vi "Execute New VI From Template.vi"(6 "Mouse Position":T2, 8 "User VI Ref":refnum<vi>, 9 "Menu Item Tag Suffix":string, 10 "Remaining Items":refnum<vi>[](array[refnum]), 11 "Affected Items":cluster{"Any Refnums":refnum<vi>[]}) -> (0 "Fail transaction?":bool)   [LabVIEW 2021]
doc: "This is the main VI of the \"New VI From Template\" shortcut menu plugin.\n\nNotes from shortcut menu template VI:\n1. This VI has no need for a Close Reference call because GObject refnums do not hold the VI in memory. The User VI Ref will be closed by the caller.\n2. You may enable debugging on this VI to help develop your code. Debugging only has to be disabled on the builder VI, not the execute VI.\n\nPetru Tarabuta, Robusto Systems, September 2022"
uses:
  <vilib>/Utility/miscctls.llb/LVPositionTypeDef.ctl
  Owner Status (enum).ctl
  GUI Objects (cluster).ctl
  Testing Flag (enum).ctl
  Testing Flag (library variable).vi
panel:
  in  "SCL":i32(listbox) caption="Templates"
  in  "Apply Owner Icon Template?":bool
  out "Error Out":errorcluster
  out "Owner Filename (including extension)":string
  out "User VI Owner Status":T1
  out "Owner Path":path
  out "Iteration":i32
  out "Tab":enum32{"SomeTemplatesFound", "NoTemplatesFound"}(tab)
  in  "Create":bool
  in  "Destination Location":path
  in  "Add To Owner?":bool caption="Add to Library 1.lvlib?"
  in  "Add To Project?":bool caption="Add to Project?"
  in  "Open Front Panel?":bool caption="Open Front Panel When Created?"
  in  "Project ComboBox":string(combo) caption="Project"
  out "NoTemplatesFound Message":string
  in  "Front Panel Sizing Tool":bool
  # "Execute VI"
  # "The section below is not user-facing. For developer use only."
  # "All controls on this panel except \"Affected Items\" have been locked to prevent accidental edits. Changing the control names or types, other than the elements of the \"Affected Items\" cluster will make the VI unusable as a menu plugin.\n\nSee Context Help for each control for details about its use."
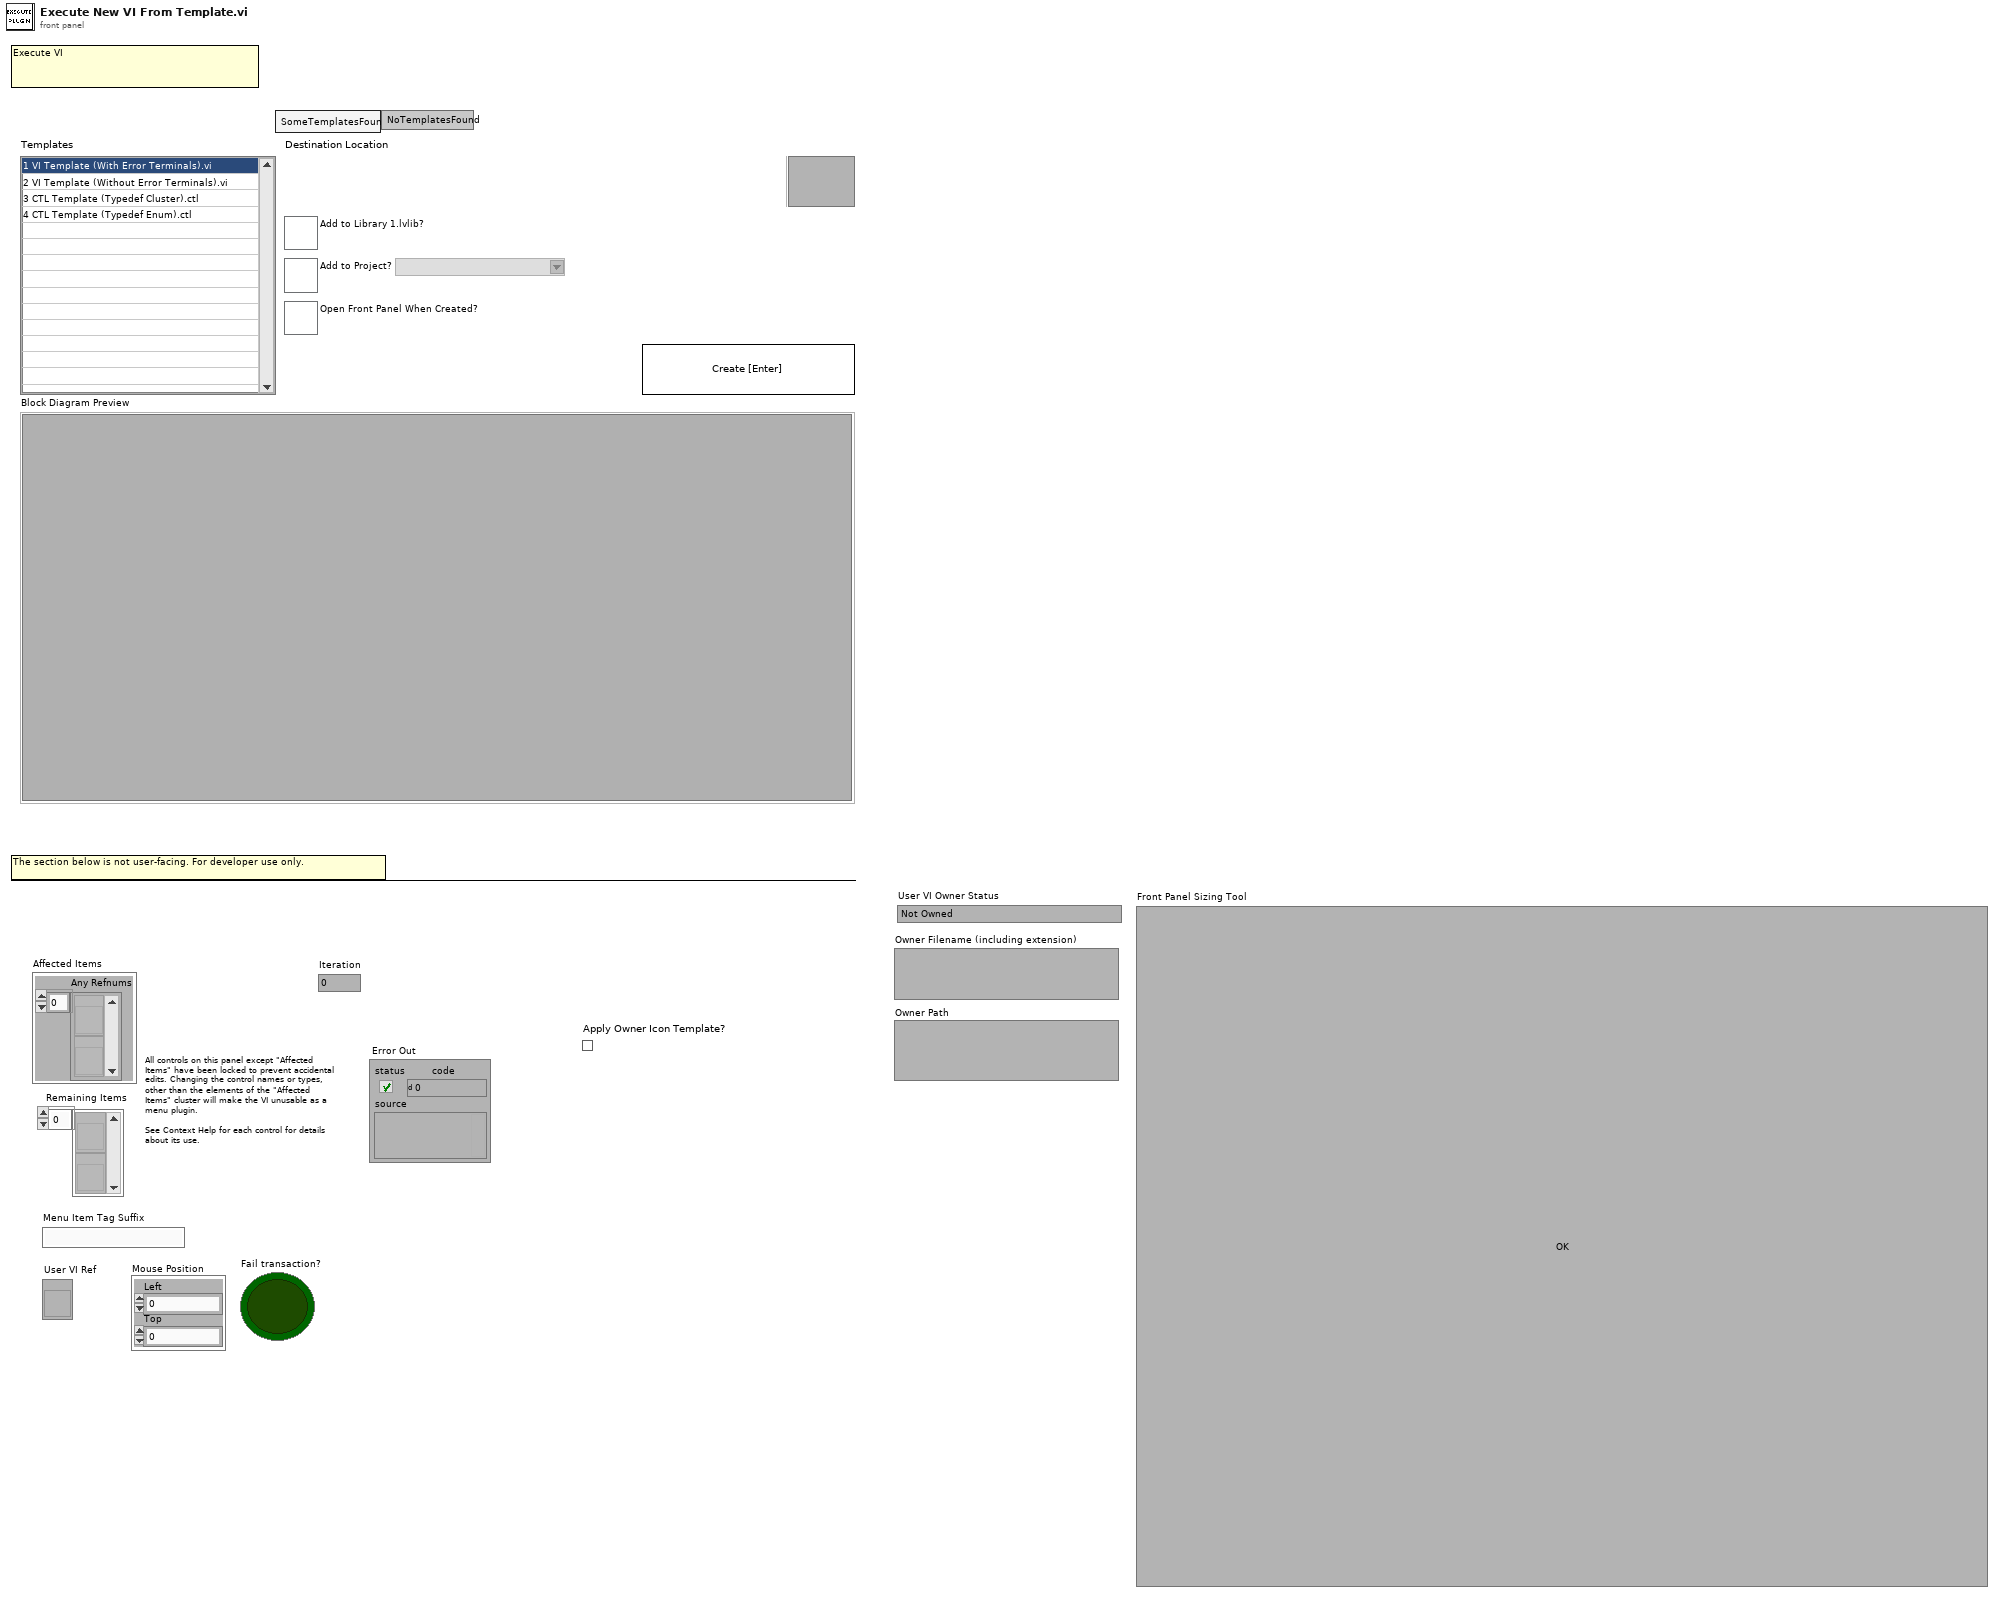
[diagram p1: front panel]
types:
  T1 = typedef "Owner Status (enum).ctl" = enum16{"Not Owned", "Owned by Library (lvlib)", "Owned by Class (lvclass)"}
  T2 = typedef "LVPositionTypeDef.ctl" = cluster{"Left":i32, "Top":i32}
  T3 = typedef "GUI Objects (cluster).ctl" = cluster{"SCL":refnum<vi>, "Add To Owner?":refnum<vi>, "Add To Project?":refnum<vi>, "Open Front Panel?":refnum<vi>, "Destination Folder":refnum<vi>, "Create":refnum<vi>, "Project ComboBox":refnum<vi>, "NoTemplatesFound Message":refnum<vi>, "Diagram Preview Subpanel":refnum<vi>}
  T4 = typedef "Testing Flag (enum).ctl" = enum16{"Production", "Testing"}
  T5 = enum32{"Invalid", "Standard", "Closed", "Hidden", "Minimized", "Maximized"}
  T6 = enum8{"Enabled", "Disabled", "Disabled and Grayed Out"}
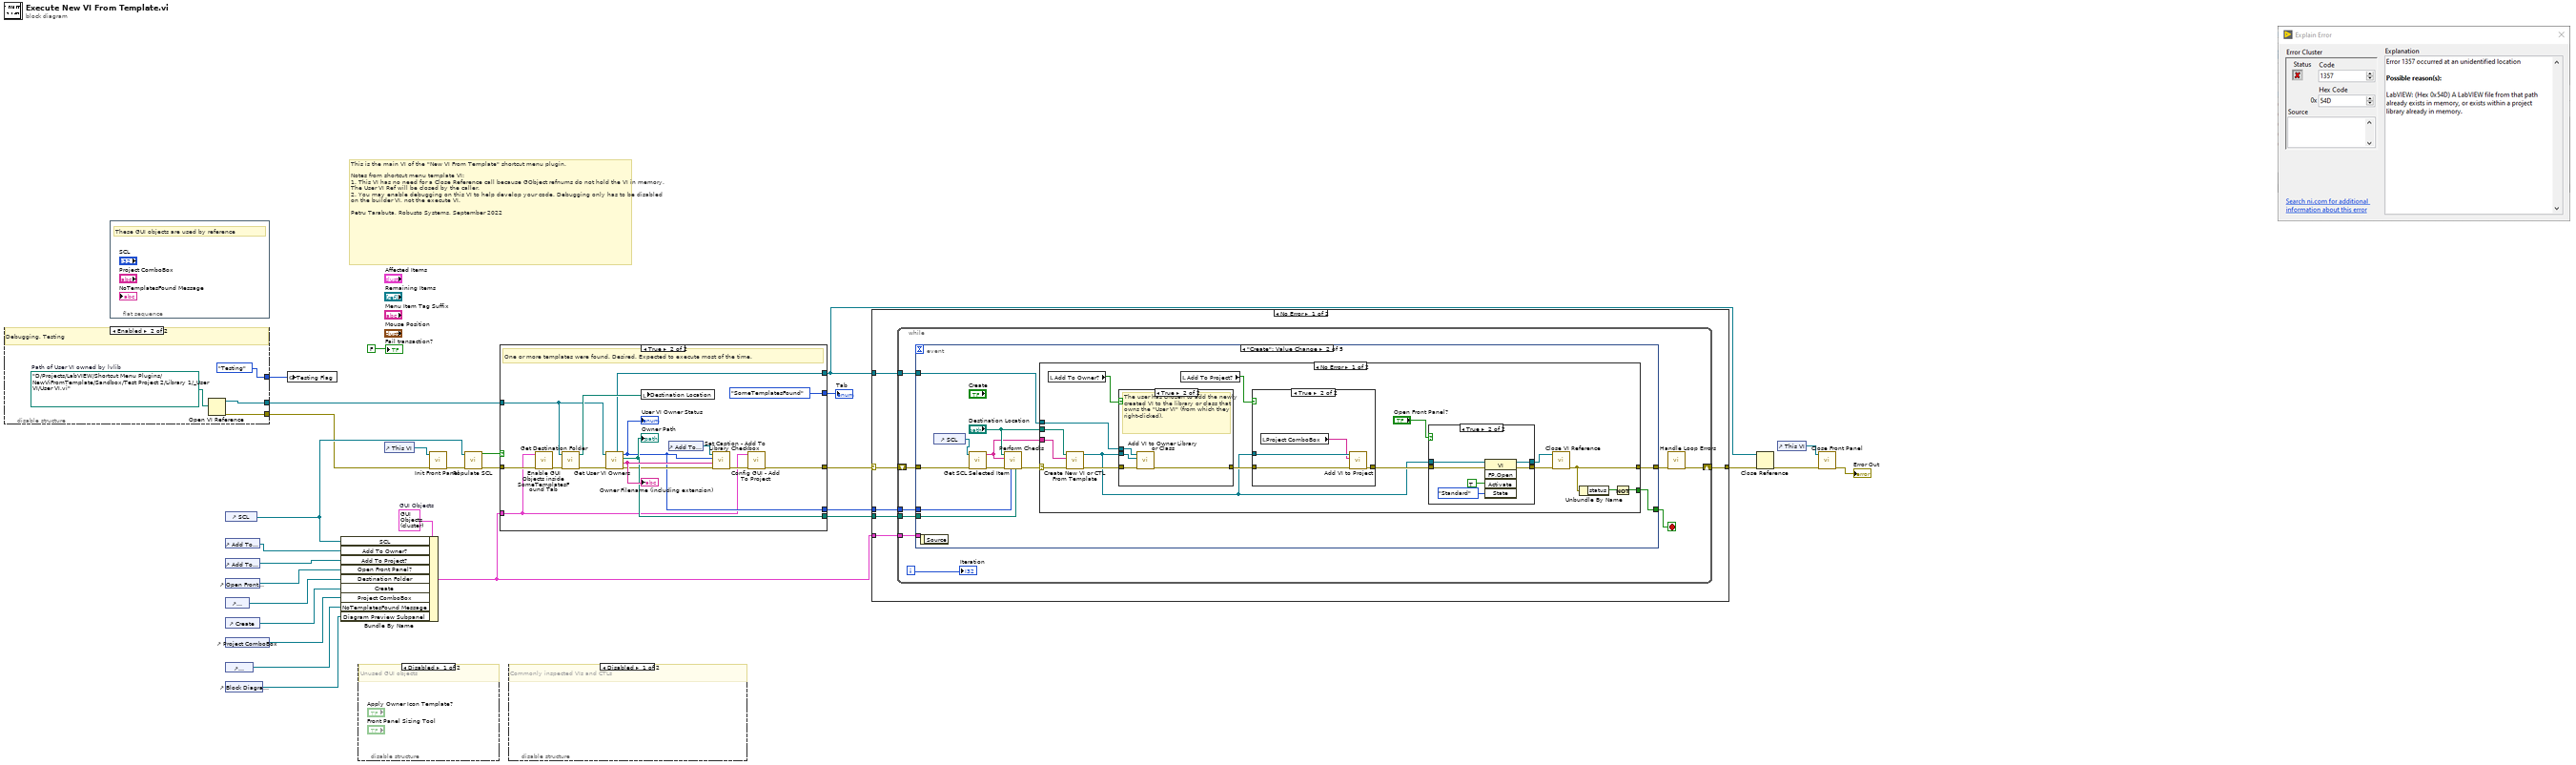
[diagram p0: block diagram]
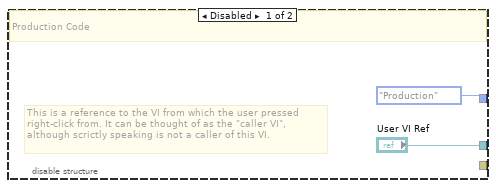
[diagram p3: hidden frame]
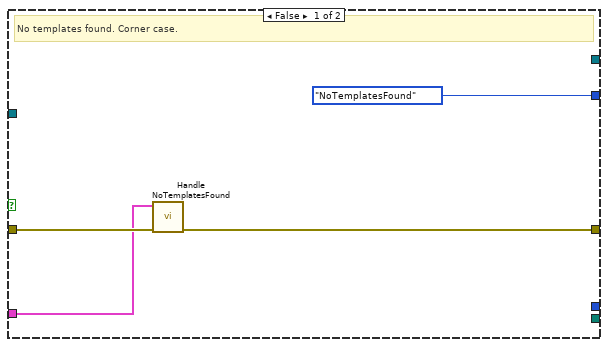
[diagram p4: hidden frame]
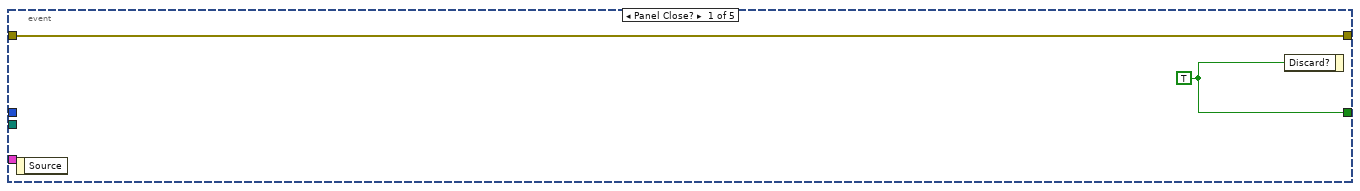
[diagram p6: hidden frame]
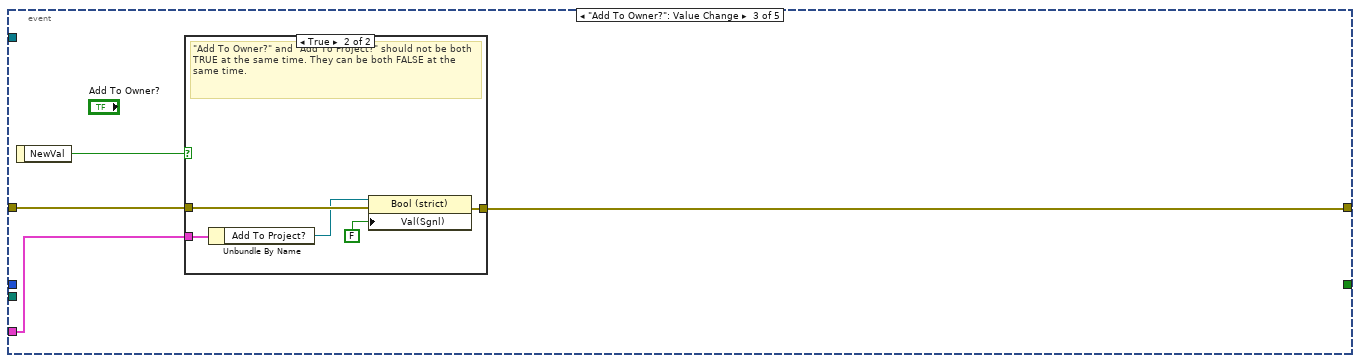
[diagram p11: hidden frame]
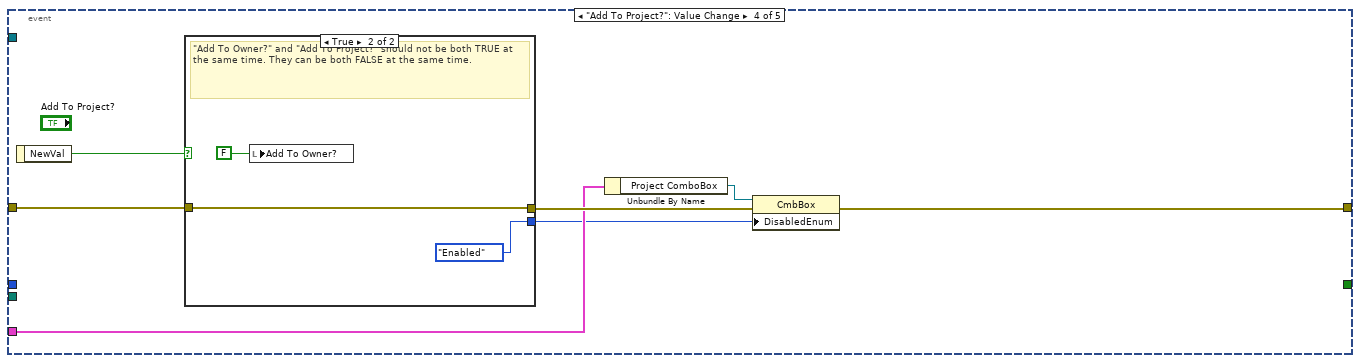
[diagram p13: hidden frame]
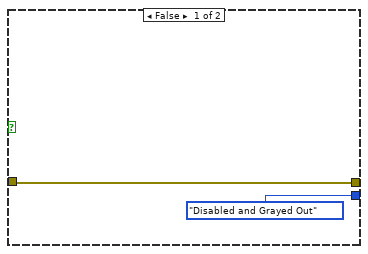
[diagram p14: hidden frame]
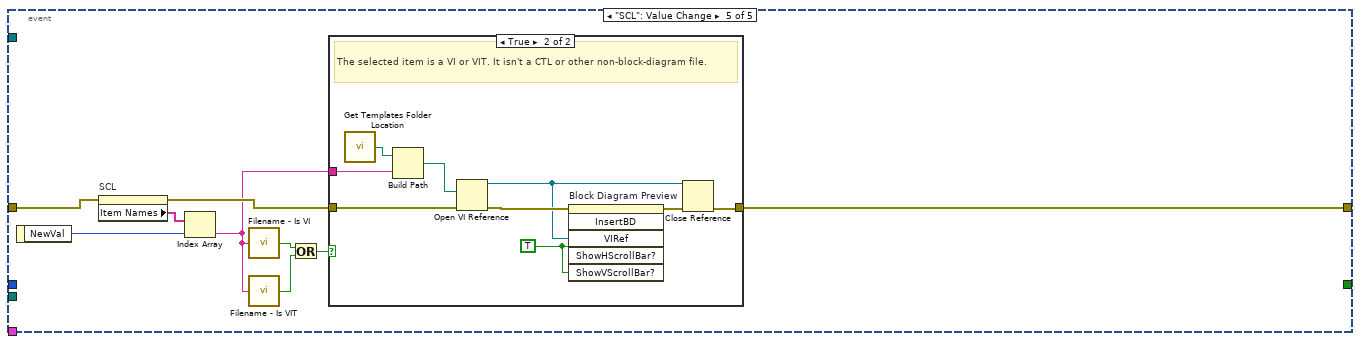
[diagram p15: hidden frame]
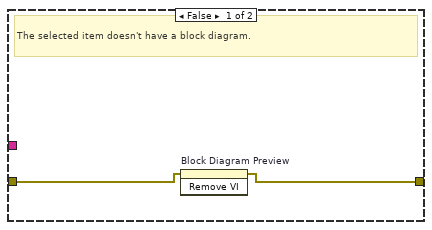
[diagram p16: hidden frame]
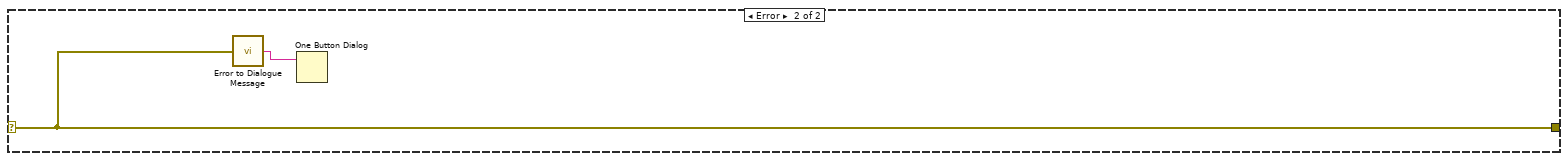
[diagram p17: hidden frame]
diagram:
  w21 = T3 {"SCL"=refnum, "Add To Owner?"=refnum, "Add To Project?"=refnum, "Open Front Panel?"=refnum, "Destination Folder"=refnum, "Create"=refnum, "Project ComboBox"=refnum, "NoTemplatesFound Message"=refnum, "Diagram Preview Subpanel"=refnum}  # GUI Objects
  # "This is the main VI of the \"New VI From Template\" shortcut menu plugin.\n\nNotes from shortcut menu template VI:\n1. This VI has no need for a Close Reference call because GObject refnums do not hold the VI in memory. The User VI Ref will be closed by the caller.\n2. You may enable debugging on this VI to help develop your code. Debugging only has to be disabled on the builder VI, not the execute VI.\n\nPetru Tarabuta, Robusto Systems, September 2022"
  n1 = disable-structure shown="Enabled" {
    disable-tunnel: ["User VI Ref" w32] -> w2
    disable-tunnel: [Testing_Flag_(enum)."Production" ("Testing Flag") Testing_Flag_(enum)."Testing" ("Testing Flag")] -> w12
    disable-tunnel: [_ w31] -> w9
    frame Disabled {
      # "This is a reference to the VI from which the user pressed right-click from. It can be thought of as the \"caller VI\", although scrictly speaking is not a caller of this VI."
      # "Production Code"
    }
    frame Enabled {
      w33 = path "D:/Projects/LabVIEW/Shortcut Menu Plugins/NewViFromTemplate/Sandbox/Test Project 2/Library 1/_User VI/User VI.vi"  # Path of User VI owned by lvlib
      # "Debugging, Testing"
      n2 = Open VI Reference(vi path=w33) -> (vi reference=w32:refnum<vi>, error out=w31:errorcluster)  [unwired: 5 in]
    }
  }
  n3 = flat-sequence {
    frame #0 {
      # "These GUI objects are used by reference"
    }
  }
  n4 = control-ref of="SCL"() -> (w20:refnum<vi>)
  n5 = control-ref of="Add To Owner?"() -> (w19:refnum<vi>)
  n6 = control-ref of="Add To Project?"() -> (w16:refnum<vi>)
  n7 = control-ref of="Open Front Panel?"() -> (w15:refnum<vi>)
  n8 = control-ref of="Destination Location"() -> (w18:refnum<vi>)
  n9 = control-ref of="Create"() -> (w17:refnum<vi>)
  n10 = control-ref of="Project ComboBox"() -> (w8:refnum<vi>)
  n11 = control-ref of="NoTemplatesFound Message"() -> (w3:refnum<vi>)
  n12 = control-ref of="Block Diagram Preview"() -> (w1:refnum<vi>)
  n13 = global write "Testing Flag (library variable).vi" "Testing Flag"(w12) -> ()
  n14 = Bundle By Name(cluster=w21, "SCL"=w20, "Add To Owner?"=w19, "Add To Project?"=w16, "Open Front Panel?"=w15, "Destination Folder"=w18, "Create"=w17, "Project ComboBox"=w8, "NoTemplatesFound Message"=w3, "Diagram Preview Subpanel"=w1) -> (w6:T3)
  n15 = disable-structure shown="Disabled" {
    frame Disabled {
      # "Unused GUI objects"
    }
    frame Enabled {
    }
  }
  n16 = control-ref of="This VI"() -> (w27:refnum<vi>)
  n17 = call "Init Front Panel.vi"("error in"=w9, "VI Reference"=w27) -> ("error out"=w26:errorcluster)  [unwired: 9 in]
  n18 = call "Populate SCL.vi"("error in"=w26, "SCL"=w20) -> ("error out"=w14:errorcluster, "At least one template file found?"=w5:bool)  [unwired: 8 in]
  n19 = case shown="True" w5 {
    tunnel: [_ w48] -> w22
    tunnel: w2 -> [_ w47]
    tunnel: w14 -> [w38 w45]
    tunnel: [_ w44] -> w13
    tunnel: [_ w43] -> w10
    tunnel: [w36 w42] -> w7
    tunnel: w6 -> [w35 w39]
    tunnel: [enum32{"SomeTemplatesFound", "NoTemplatesFound"}."NoTemplatesFound" ("Tab") enum32{"SomeTemplatesFound", "NoTemplatesFound"}."SomeTemplatesFound" ("Tab")] -> w4
    frame False {
      # "No templates found. Corner case."
      n20 = call "Handle NoTemplatesFound.vi"("error in"=w38, "GUI Objects"=w35) -> ("error out"=w36:errorcluster)  [unwired: 9 in]
    }
    frame True {
      # "One or more templates were found. Desired. Expected to execute most of the time."
      n21 = call "Enable GUI Objects inside SomeTemplatesFound Tab.vi"("error in"=w45, "GUI Objects"=w39) -> ("error out"=w40:errorcluster)  [unwired: 9 in]
      n22 = call "Get Destination Folder.vi"("error in"=w40, "User VI Ref"=w47) -> ("error out"=w53:errorcluster, "Destination Folder"=w49:path)  [unwired: 8 in]
      n23 = call "Get User VI Owners.vi"("error in"=w53, "User VI Ref"=w47) -> ("error out"=w46:errorcluster, "Owner Filename (inc file extension)"=w50:string, "Owner Path"=w48:path, "User VI Owner Status"=w44:T1, "Owner Reference"=w43:refnum<vi>)  [unwired: 4 in, 1 out]
      "Owner Path" <- w48
      "User VI Owner Status" <- w44
      "Owner Filename (including extension)" <- w50
      n24 = local write "Destination Location"(w49) -> ()
      n25 = control-ref of="Add To Owner?"() -> (w51:refnum<vi>)
      n26 = call "Set Caption - Add To Library Checkbox.vi"("error in"=w46, "Owner Filename (including extension)"=w50, "User VI Owner Status"=w44, "Add To Owner"=w51) -> ("error out"=w52:errorcluster)  [unwired: 7 in]
      n27 = call "Config GUI - Add To Project.vi"("error in"=w52, "GUI Objects"=w39) -> ("error out"=w42:errorcluster)  [unwired: 8 in, 1 out]
    }
  }
  "Tab" <- w4
  n28 = disable-structure shown="Disabled" {
    frame Disabled {
      # "Commonly inspected VIs and CTLs"
    }
    frame Enabled {
    }
  }
  n29 = case shown="No Error" w7 {
    selector: w7 -> [w59 w160]
    tunnel: [w58 w160] -> w25
    tunnel: w13 -> [w57 _]
    tunnel: w22 -> [w56 _]
    tunnel: w6 -> [w55 _]
    tunnel: w10 -> [w54 _]
    frame No Error {
      n30 = while {
        shift-right: [w62] -> w58
        shift-left: w59 -> [w68]
        tunnel: w57 -> [w65]
        tunnel: w56 -> [w64]
        tunnel: w55 -> [w61]
        tunnel: w54 -> [w60]
        i -> [w67]
        stop <- w66 stop-if-true
        n31 = event shown="[1] \"Create\": Value Change" {
          selector: _ -> [_ _ _ _ _]
          dyn-events: _ -> [_ _ _ _ _]
          timeout: _ -> [_ _ _ _ _]
          tunnel: w68 -> [w69 w80 w119 w132 w147]
          tunnel: [w70 w72 _ _ _] -> w66
          tunnel: [w69 w81 w118 w130 w141] -> w63
          tunnel: w65 -> [_ w77 _ _ _]
          tunnel: w64 -> [_ w76 _ _ _]
          tunnel: w61 -> [_ _ w117 w129 _]
          tunnel: w60 -> [_ w73 _ _ _]
          event Panel Close? {
            w70 = TRUE
            n32 = event-data() -> ()  [unwired: 1 in, 1 out]
            n33 = event-data("Discard?"=w70) -> ()  [unwired: 1 in, 1 out]
          }
          event "Create": Value Change {
            n34 = event-data() -> ()  [unwired: 1 in, 1 out]
            n35 = control-ref of="SCL"() -> (w71:refnum<vi>)
            n36 = call "Get SCL Selected Item.vi"("error in"=w80, "SCL"=w71) -> ("error out"=w79:errorcluster, "Selected Item (String)"=w74:string)  [unwired: 7 in, 1 out]
            n37 = call "Perform Checks.vi"("Owner Path (if applicable)"=w76, "User VI Owner Status"=w77, "error in"=w79, "Selected Template VI or CTL name (including file extension)"=w74, "Destination Folder"="Destination Location") -> ("error out"=w78:errorcluster)  [unwired: 6 in]
            n38 = case shown="No Error" w78 {
              selector: w78 -> [w97 w116]
              tunnel: [w84 w116] -> w81
              tunnel: "Destination Location" -> [w96 _]
              tunnel: w74 -> [w95 _]
              tunnel: w73 -> [w92 _]
              tunnel: [w82 _] -> w72
              frame No Error {
                n39 = local read "Add To Owner?"() -> (w94:bool)
                n40 = call "Create New VI or CTL From Template.vi"("error in"=w97, "Selected Template VI or CTL name (including file extension)"=w95, "Destination Folder"=w96) -> ("error out"=w93:errorcluster, "Reference of newly created VI"=w85:refnum<vi>)  [unwired: 7 in]
                n41 = case shown="True" w94 {
                  tunnel: [w103 w107] -> w88
                  tunnel: w93 -> [w103 w106]
                  tunnel: w85 -> [_ w105]
                  tunnel: w92 -> [_ w104]
                  frame False {
                  }
                  frame True {
                    # "The user has chosen to add the newly created VI to the library or class that owns the \"User VI\" (from which they right-clicked)."
                    n42 = call "Add VI to Owner Library or Class.vi"("error in"=w106, "Reference of newly created VI"=w105, "Owner Reference (Library or Class)"=w104) -> ("error out"=w107:errorcluster)  [unwired: 8 in]
                  }
                }
                n43 = local read "Add To Project?"() -> (w86:bool)
                n44 = case shown="True" w86 {
                  tunnel: [w98 w102] -> w87
                  tunnel: w88 -> [w98 w101]
                  tunnel: w85 -> [_ w100]
                  frame False {
                  }
                  frame True {
                    n45 = local read "Project ComboBox"() -> (w99:string)
                    n46 = call "Add VI to Project.vi"("error in"=w101, "Add VI to this Project"=w99, "Reference of newly created VI or CTL"=w100) -> ("error out"=w102:errorcluster)  [unwired: 8 in]
                  }
                }
                n47 = case shown="True" "Open Front Panel?" {
                  tunnel: w87 -> [w109 w115]
                  tunnel: [w109 w114] -> w91
                  tunnel: w85 -> [w108 w113]
                  tunnel: [w108 w110] -> w90
                  frame False {
                  }
                  frame True {
                    n48 = invoke class="VI" method="FP.Open"(reference=w113, error in=w115, "Activate"=TRUE ("Activate?"), "State"=T5."Standard") -> (reference out=w110:refnum<vi>, error out=w114:errorcluster)  [unwired: 1 in, 3 out]
                  }
                }
                n49 = call "Close VI Reference.vi"("error in"=w91, "VI Reference"=w90) -> ("error out"=w84:errorcluster)  [unwired: 9 in]
                n50 = Unbundle By Name(w84) -> ("status"=w83:bool)
                n51 = Not(x=w83) -> (.not. x?=w82:bool)
              }
              frame Error {
              }
            }
          }
          event "Add To Owner?": Value Change {
            n52 = event-data() -> ("NewVal"=w120:bool)  [unwired: 1 in]
            n53 = case shown="True" w120 {
              tunnel: w119 -> [w121 w126]
              tunnel: [w121 w125] -> w118
              tunnel: w117 -> [_ w124]
              frame False {
              }
              frame True {
                # "\"Add To Owner?\" and \"Add To Project?\" should not be both TRUE at the same time. They can be both FALSE at the same time."
                n54 = Unbundle By Name(w124) -> ("Add To Project?"=w123:refnum<vi>)
                n55 = property class="Bool (strict)"(reference=w123, error in=w126, "Val(Sgnl)"=FALSE ("Value (Signaling)")) -> (error out=w125:errorcluster)  [unwired: 1 out]
              }
            }
          }
          event "Add To Project?": Value Change {
            n56 = event-data() -> ("NewVal"=w133:bool)  [unwired: 1 in]
            n57 = case shown="True" w133 {
              tunnel: w132 -> [w135 w137]
              tunnel: [w135 w137] -> w131
              tunnel: [T6."Disabled and Grayed Out" ("Disabled") T6."Enabled" ("Disabled")] -> w127
              frame False {
              }
              frame True {
                # "\"Add To Owner?\" and \"Add To Project?\" should not be both TRUE at the same time. They can be both FALSE at the same time."
                n58 = local write "Add To Owner?"(FALSE ("Add To Project?")) -> ()
              }
            }
            n59 = Unbundle By Name(w129) -> ("Project ComboBox"=w128:refnum<vi>)
            n60 = property class="CmbBox"(reference=w128, error in=w131, "DisabledEnum"=w127) -> (error out=w130:errorcluster)  [unwired: 1 out]
          }
          event "SCL": Value Change {
            n61 = event-data() -> ("NewVal"=w145:i32)  [unwired: 1 in]
            n62 = property on="SCL" class="LstBox (strict)"(error in=w147) -> (error out=w142:errorcluster, "Item Names"=w146:string[])  [unwired: 1 in, 1 out]
            n63 = Index Array(array=w146, index=w145) -> (element=w139:string)
            n64 = call "Filename - Is VI.vi"("Filename (including file extension)"=w139) -> ("Is VI?"=w143:bool)
            n65 = call "Filename - Is VIT.vi"("Filename (including file extension)"=w139) -> ("Is VIT?"=w144:bool)
            n66 = Or(x=w143, y=w144) -> (x .or. y?=w140:bool)
            n67 = case shown="True" w140 {
              tunnel: w142 -> [w148 w158]
              tunnel: [w149 w151] -> w141
              tunnel: w139 -> [_ w156]
              frame False {
                # "The selected item doesn't have a block diagram."
                n68 = invoke on="Block Diagram Preview" class="SubPnl" method="Remove VI"(error in=w148) -> (error out=w149:errorcluster)  [unwired: 2 in, 2 out]
              }
              frame True {
                w154 = TRUE ("ShowHScrollBar")
                # "The selected item is a VI or VIT. It isn't a CTL or other non-block-diagram file."
                n69 = call "Get Templates Folder Location.vi"() -> ("Templates Folder Location"=w157:path)
                n70 = Build Path(base path=w157, name or relative path=w156) -> (appended path=w155:path)
                n71 = Open VI Reference(vi path=w155, error in (no error)=w158) -> (vi reference=w150:refnum<vi>, error out=w153:errorcluster)  [unwired: 4 in]
                n72 = invoke on="Block Diagram Preview" class="SubPnl" method="InsertBD"(error in=w153, "VIRef"=w150, "ShowHScrollBar?"=w154, "ShowVScrollBar?"=w154) -> (error out=w152:errorcluster)  [unwired: 2 in, 5 out]
                n73 = Close Reference(reference=w150, error in (no error)=w152) -> (error out=w151:errorcluster)
              }
            }
          }
        }
        n74 = call "Handle Loop Errors.vi"("error in"=w63) -> ("error out"=w62:errorcluster)  [unwired: 10 in]
        "Iteration" <- w67
      }
    }
    frame Error {
      n75 = call "Error to Dialogue Message.vi"("error in"=w160) -> ("Dialogue Message"=w159:string)
      n76 = One Button Dialog(message=w159) -> ()  [unwired: 1 in, 1 out]
    }
  }
  n77 = Close Reference(reference=w10, error in (no error)=w25) -> (error out=w11:errorcluster)
  n78 = control-ref of="This VI"() -> (w24:refnum<vi>)
  n79 = call "Close Front Panel.vi"("error in"=w11, "VI Reference"=w24) -> ("error out"=→"Error Out":errorcluster)  [unwired: 9 in]
  "Fail transaction?" <- FALSE ("Fail transaction?")
